vi "SLL DE DO Intercon Lines.vi"(8 "Error In":errorcluster) -> (0 "Error Out":errorcluster, 3 "DO Name":T1[][](array[typedef]))   [LabVIEW 2013]
doc: "Copyright © 2005, Soliton Technologies.\nAll rights reserved."
uses:
  Controls/SLL DE List of Digital Outputs.ctl
  Controls/SLL DE DAQ Parameters LV2Global Options.ctl
  Instance           1 32Saved   SLL DE DO Intercon Lines .vi
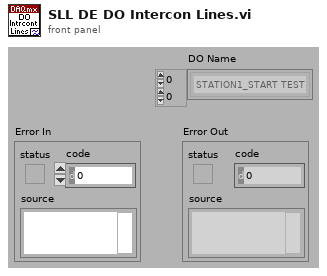
[diagram p1: front panel]
types:
  T1 = typedef "SLL DE List of Digital Outputs.ctl" = enum16{"STATION1_START TEST", "STATION1_STOP TEST", "STATION1_LIGHT1", "STATION1_LIGHT2", "STATION1_LIGHT3", "STATION2_START TEST", "STATION2_STOP TEST", "STATION2_LIGHT1", "STATION2_LIGHT2", "STATION2_LIGHT3", "STATION3_START TEST", "STATION3_STOP TEST", "STATION3_LIGHT1", "STATION3_LIGHT2", "STATION3_LIGHT3", "STATION4_START TEST", "STATION4_STOP TEST", "STATION4_LIGHT1", "STATION4_LIGHT2", "STATION4_LIGHT3"}
  T2 = typedef "SLL DE DAQ Parameters LV2Global Options.ctl" = enum16{"Read", "Write"}
  T3 = typedef "SLL DE DAQ Engine Parameters.ctl" = cluster{"Enable Engines":cluster{"AI Enable":bool, "AO Enable":bool, "DI Enable":bool, "DO Enable":bool}, "DAQ Control Type":cluster{"Analog Input":enum16{"Finite", "Continuous", "Driver"}, "Analog Output":enum16{"Finite", "Continuous", "Driver"}, "Digital Input":enum16{"Finite", "Continuous", "Driver"}, "Digital Output":enum16{"Finite", "Continuous", "Driver"}}, "DAQ Parameters":cluster{"AI Sampling Rate (Samples/Sec)":dbl, "MvgAVG Window Size (# of Points)":i32, "Enable Filter":bool, "Enable MvgAVG":bool, "Circular Buffer Size (Sec)":dbl, "AO Sampling Rate (Samples/Sec)":dbl, "Graph Update Rate (Samples/Sec)":dbl, "File Logging Rate (Samples/Sec)":i32}, "AO Safe Values":cluster{"Analog Outputs Name":T4, "Analog Outputs Safe Value":dbl}[], "DO Safe Values":cluster{"Digital Outputs Name":T1, "Digital Outputs Safe Value":bool}[], "DO Interconnected Lines":cluster{"First DO Line":string, "Second DO Line":string}[], "AI Channels Unit":cluster{"Channel Name":T5, "Channel Type":T6}[], "Units Information":cluster{"Channel Type":T6, "Unit Text":string, "Maximum":dbl, "Minmum":dbl, "Increments":dbl}[]}
  T4 = typedef "SLL DE List of Analog Outputs.ctl" = enum16{"None"}
  T5 = typedef "SLL DE List of Analog Inputs.ctl" = enum16{"None"}
  T6 = typedef "SLL DE List of AI Channel Type.ctl" = enum16{"Pressure", "Flow", "Temperature", "Time Scale", "Voltage", "Current", "Frequency", "Sound", "Speed", "Torque", "Distance", "Channel Type 1", "Channel Type 2", "Channel Type 3"}
  T7 = cluster{"First DO Line":string, "Second DO Line":string}[]
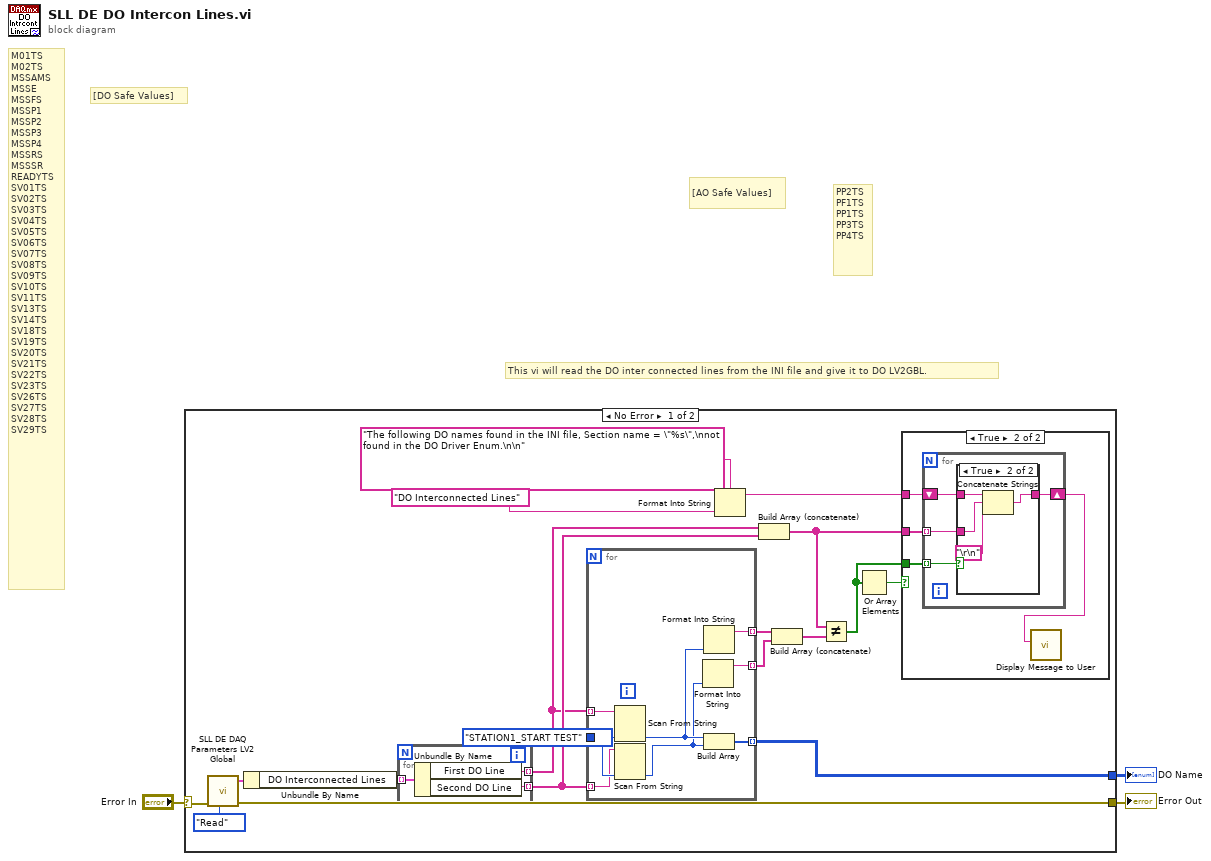
[diagram p0: block diagram]
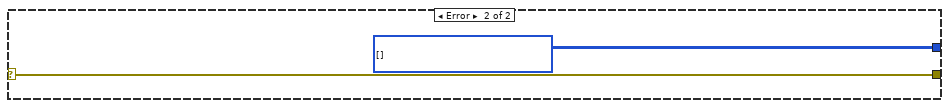
[diagram p4: hidden frame]
diagram:
  # "This vi will read the DO inter connected lines from the INI file and give it to DO LV2GBL."
  # "[DO Safe Values]"
  # "PP2TS\nPF1TS\nPP1TS\nPP3TS\nPP4TS"
  # "[AO Safe Values]"
  # "M01TS\nM02TS\nMSSAMS\nMSSE\nMSSFS\nMSSP1\nMSSP2\nMSSP3\nMSSP4\nMSSRS\nMSSSR\nREADYTS\nSV01TS\nSV02TS\nSV03TS\nSV04TS\nSV05TS\nSV06TS\nSV07TS\nSV08TS\nSV09TS\nSV10TS\nSV11TS\nSV13TS\nSV14TS\nSV18TS\nSV19TS\nSV20TS\nSV21TS\nSV22TS\nSV23TS\nSV26TS\nSV27TS\nSV28TS\nSV29TS"
  n1 = case shown="No Error" "Error In" {
    selector: "Error In" -> [w8 w47]
    tunnel: [w7 w47] -> w2
    tunnel: [w4 w46] -> w1
    frame No Error {
      n2 = call "SLL DE DAQ Parameters LV2 Global.vi"("Option"=SLL_DE_DAQ_Parameters_LV2Global_Options."Read", "Error in (no error)"=w8) -> ("Error out"=w7:errorcluster, "Global Info"=w10:T3)  [unwired: 8 in]
      n3 = Unbundle By Name(w10) -> ("DO Interconnected Lines"=w11:T7)
      n4 = for {
        tunnel: w11 -> [w24] mode=indexing
        tunnel: [w23] -> w5 mode=indexing
        tunnel: [w22] -> w6 mode=indexing
        n5 = Unbundle By Name(w24) -> ("First DO Line"=w23:string, "Second DO Line"=w22:string)
      }
      n6 = for {
        tunnel: w5 -> [w45] mode=indexing
        tunnel: SLL_DE_List_of_Digital_Outputs."STATION1_START TEST" ("List of Digital Outputs") -> [w44]
        tunnel: w6 -> [w43] mode=indexing
        tunnel: [w42] -> w4 mode=indexing
        tunnel: [w40] -> w17 mode=indexing
        tunnel: [w38] -> w16 mode=indexing
        n7 = Scan From String(input string=w45, default 1=w44) -> (output 1=w41:T1)  [unwired: 3 in, 3 out]
        n8 = Scan From String(input string=w43, default 1=w44) -> (output 1=w39:T1)  [unwired: 3 in, 3 out]
        n9 = Format Into String(w39) -> (resulting string=w38:string)  [unwired: 3 in, 1 out]
        n10 = Format Into String(w41) -> (resulting string=w40:string)  [unwired: 3 in, 1 out]
        n11 = Build Array(w41, w39) -> (w42:T1[])
      }
      n12 = Format Into String(format string="The following DO names found in the INI file, Section name = \"%s\",\nnot found in the DO Driver Enum.\n\n" ("Message"), "DO Interconnected Lines" ("Section")) -> (resulting string=w19:string)  [unwired: 2 in, 1 out]
      n13 = Build Array (concatenate)(w5, w6) -> (w12:string[])
      n14 = Build Array (concatenate)(w17, w16) -> (w15:string[])
      n15 = Not Equal?(x=w12, y=w15) -> (x != y?=w13:bool[])
      n16 = Or Array Elements(Boolean array=w13) -> (logical OR=w14:bool)
      n17 = case shown="True" w14 {
        tunnel: w19 -> [_ w28]
        tunnel: w13 -> [_ w26]
        tunnel: w12 -> [_ w25]
        frame False {
        }
        frame True {
          n18 = for {
            tunnel: w25 -> [w32] mode=indexing
            shift-right: [w30] -> w27
            shift-left: w28 -> [w31]
            tunnel: w26 -> [w29] mode=indexing
            n19 = case shown="True" w29 {
              tunnel: w32 -> [_ w37]
              tunnel: w31 -> [w33 w36]
              tunnel: [w33 w34] -> w30
              frame False {
              }
              frame True {
                n20 = Concatenate Strings(w36, w37, "\r\n") -> (w34:string)
              }
            }
          }
          n21 = call "Display Message to User"("Message"=w27) -> ()  [unwired: 9 in, 2 out]
        }
      }
    }
    frame Error {
      w46 = T1[][] [] items=["STATION1_START TEST", "STATION1_STOP TEST", "STATION1_LIGHT1", "STATION1_LIGHT2", "STATION1_LIGHT3", "STATION2_START TEST", "STATION2_STOP TEST", "STATION2_LIGHT1", "STATION2_LIGHT2", "STATION2_LIGHT3", "STATION3_START TEST", "STATION3_STOP TEST", "STATION3_LIGHT1", "STATION3_LIGHT2", "STATION3_LIGHT3", "STATION4_START TEST", "STATION4_STOP TEST", "STATION4_LIGHT1", "STATION4_LIGHT2", "STATION4_LIGHT3"]
    }
  }
  "Error Out" <- w2
  "DO Name" <- w1
